vi "DataStream_PC_Build Graph Data.vi"(11 "Map":map{string, T1}(c390)) -> (2 "Graph Data Out":cluster{"Array":dbl[], "Array":dbl[]}[](array[cluster]), 3 "Name Array Out":string[](array[string]))   [LabVIEW 2020]
uses:
  TypeDefs/Cluster_DataStream PC Map Data Set.ctl
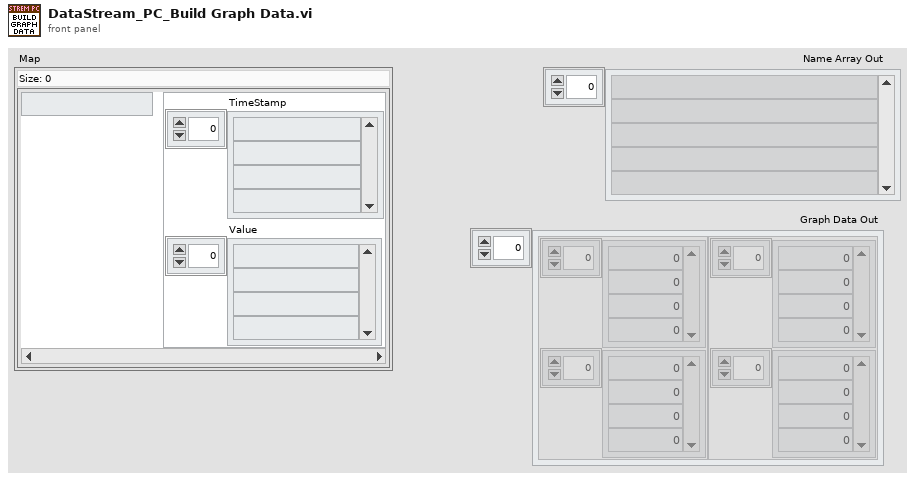
[diagram p1: front panel]
types:
  T1 = typedef "Cluster_DataStream PC Map Data Set.ctl" = cluster{"TimeStamp":dbl[], "Value":dbl[]}
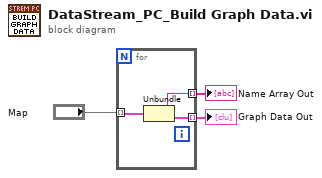
[diagram p0: block diagram]
diagram:
  n1 = for {
    tunnel: "Map" -> [w6] mode=indexing
    tunnel: [w4] -> w3 mode=indexing
    tunnel: [w5] -> w1 mode=indexing
    n2 = Unbundle(w6) -> (w5:string, w4:T1)
  }
  "Graph Data Out" <- w3
  "Name Array Out" <- w1
